vi "DHE_SetDetXYSize.vi"(2 "DHE_DetXSize":i32, 3 "DHE_DetYSize":i32) -> ()   [LabVIEW 2016]
uses:
  private/vis/DHE_GBLDriverVariables.vi
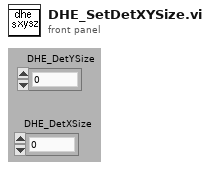
[diagram p1: front panel]
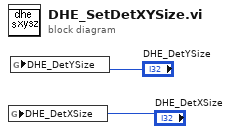
[diagram p0: block diagram]
diagram:
  n1 = global write "DHE_GBLDriverVariables.vi" "DHE_DetXSize"("DHE_DetXSize") -> ()
  n2 = global write "DHE_GBLDriverVariables.vi" "DHE_DetYSize"("DHE_DetYSize") -> ()
